vi "Command_DriveDistanceAtAngle.vi"(7 "Parameters":dbl[](array[numeric]), 11 "Startup":bool) -> (4 "Completed":bool, 6 "Target_Drive_Powers":dbl[](array[numeric]), 10 "Target_Wheel_Angles":dbl[](array[numeric]), 15 "Reinit":bool)   [LabVIEW 2020]
uses:
  Auto Utilities/Command_Execution_State.ctl
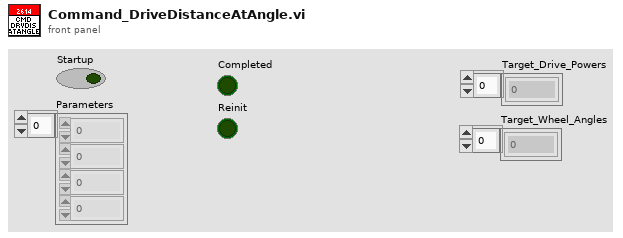
[diagram p1: front panel]
types:
  T1 = typedef "Command_Execution_State.ctl" = enum16{"Initialize", "Execute", "Finish"}
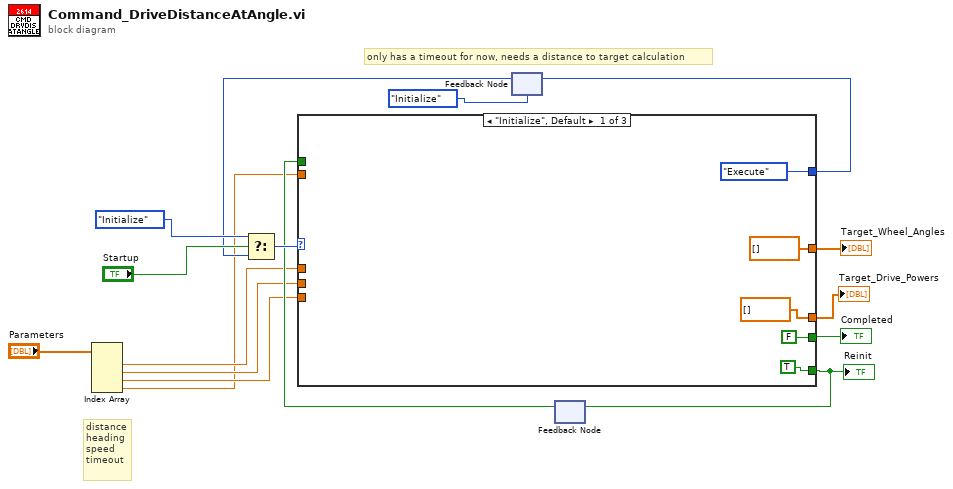
[diagram p0: block diagram]
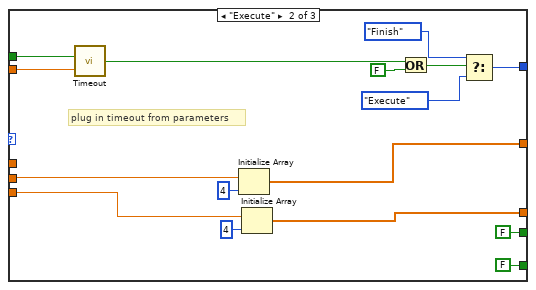
[diagram p2: hidden frame]
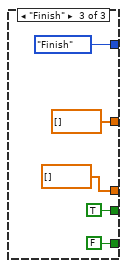
[diagram p3: hidden frame]
diagram:
  # "only has a timeout for now, needs a distance to target calculation"
  # "distance\nheading\nspeed\ntimeout"
  n1 = Index Array(array="Parameters") -> (element #1=w6:dbl, element #2=w5:dbl, element #3=w4:dbl, element #4=w3:dbl)  [unwired: 4 in]
  n2 = feedback #1(Command_Execution_State."Initialize") -> (w12:T1)
  n3 = Select(t=Command_Execution_State."Initialize", s="Startup", f=w12) -> (s? t:f=w14:T1)
  n4 = feedback #2() -> (w8:bool)  [unwired: 1 in]
  n5 = case shown="\"Initialize\", Default" w14 {
    tunnel: [Command_Execution_State."Execute" w35 Command_Execution_State."Finish"] -> w13
    tunnel: [FALSE ("Reinit") FALSE ("Reinit") TRUE ("Reinit")] -> w10
    tunnel: [TRUE ("Reinit") FALSE ("Reinit") FALSE ("Reinit")] -> w9
    tunnel: w8 -> [_ w32 _]
    tunnel: w6 -> [_ _ _]
    tunnel: w5 -> [_ w28 _]
    tunnel: w4 -> [_ w24 _]
    tunnel: w3 -> [_ w29 _]
    tunnel: [dbl[] [] w26 dbl[] []] -> w2
    tunnel: [dbl[] [] w23 dbl[] []] -> w1
    frame "Initialize", Default {
    }
    frame "Execute" {
      # "plug in timeout from parameters"
      n6 = call "Timeout.vi"("Timeout"=w29, "Initialize"=w32) -> ("Timed Out?"=w30:bool)
      n7 = Initialize Array(w28, 4 ("dimension size")) -> (w26:dbl[])
      n8 = Initialize Array(w24, 4 ("dimension size")) -> (w23:dbl[])
      n9 = Or(x=w30, y=FALSE) -> (x .or. y?=w31:bool)
      n10 = Select(t=Command_Execution_State."Finish", s=w31, f=Command_Execution_State."Execute") -> (s? t:f=w35:T1)
    }
    frame "Finish" {
    }
  }
  "Reinit" <- w9
  "Completed" <- w10
  "Target_Wheel_Angles" <- w2
  "Target_Drive_Powers" <- w1
  n11 = feedback-in #1(w13) -> ()
  n12 = feedback-in #2(w9) -> ()
